vi "SourceAllOff.vi"(3 "Source":string="PI1-MAGLITE", 9 "error in (no error)":errorcluster) -> (0 "Source out":string="PI1-MAGLITE", 1 "Ok?":refnum<k4>, 6 "error out":errorcluster)   [LabVIEW 2009]
uses:
  Controls/SourceCommand.ctl
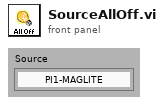
[diagram p1: front panel]
types:
  T1 = typedef "SourceCommand.ctl" = cluster{"Source":string, "Command":enum16{"INTENSITY", "ALL OFF", "QUIT"}, "Intensity":i32, "Ok?":refnum<k4>}
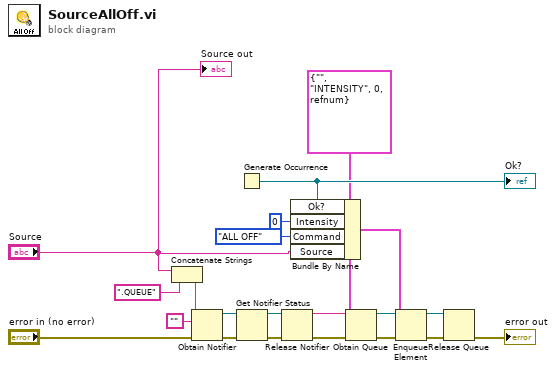
[diagram p0: block diagram]
diagram:
  w12 = T1 {"Source"="", "Command"=enum."INTENSITY", "Intensity"=0, "Ok?"=refnum} ("SourceCommand")
  n1 = Concatenate Strings("Source", ".QUEUE") -> (w6:string)
  n2 = Obtain Notifier(name (unnamed)=w6, notification data type="", error in (no error)="error in (no error)") -> (notifier out=w7:refnum<notifier>, error out=w8:errorcluster)  [unwired: 1 in, 1 out]
  n3 = Generate Occurrence() -> (w15:refnum<k4>)
  "Ok?" <- w15
  n4 = Get Notifier Status(notifier=w7, error in (no error)=w8) -> (notifier out=w10:refnum<notifier>, error out=w11:errorcluster)  [unwired: 3 out]
  n5 = Release Notifier(notifier=w10, error in (no error)=w11) -> (notifier name=w2:string, error out=w1:errorcluster)  [unwired: 2 out]
  n6 = Bundle By Name(cluster=w12, "Ok?"=w15, "Intensity"=0, "Command"=enum16{"INTENSITY", "ALL OFF", "QUIT"}."ALL OFF", "Source"="Source") -> (w19:T1)
  n7 = Obtain Queue(name (unnamed)=w2, element data type=w12, error in (no error)=w1) -> (queue out=w21:refnum<queue>, error out=w20:errorcluster)  [unwired: 2 in, 1 out]
  n8 = Enqueue Element(queue=w21, element=w19, error in (no error)=w20) -> (queue out=w16:refnum<queue>, error out=w18:errorcluster)  [unwired: 2 out]
  n9 = Release Queue(queue=w16, error in (no error)=w18) -> (error out=→"error out":errorcluster)  [unwired: 3 out]
  "Source out" <- "Source"
